vi "fgv_NtripClient_config.vi"(7 "cmd":T2, 11 "config val":T1={"Current NtripClient Account"={"id"="seoul", "pwd"="seoul", "ref pt"="YONS-RTCM32-M5", "address"="gnss.eseoul.go.kr", "port "=2101}, "Mount points"=0, "Ref r size"=1.0, "TMarr limit"=200, "Sel NMEA type"=enum."$GPGGA", "Local Time offset"=9, "Write delay ms"=900, "GNSS Serial delay"=20, "Extra Serial delay"=20, "Ntrip accounts"=[], "Send Serial config"={"NMEA out port"="COM10", "baud rate"=115200}} {"Ref r size" format="%.2f"; "Mount points" items=["SONP-RTCM32", "GANS-RTCM32", "GUMC-RTCM32", "DBON-RTCM32", "YONS-RTCM23", "SONP-RTCM23", "GUMC-RTCM23", "GANS-RTCM31", "YONS-CMRx", "SONP-RTCM31", "GUMC-RTCM31", "GANS-RTCM23", "DBON-RTCM23", "DBON-RTCM31", "YONS-RTCM31", "YONS-RTCM32-M5", "VRS-RTCM32-M5", "VRS-RTCM31", "VRS-CMRx", "VRS-CMRplus"]}) -> (3 "config val out":T1={"Current NtripClient Account"={"id"="seoul", "pwd"="seoul", "ref pt"="YONS-RTCM32-M5", "address"="gnss.eseoul.go.kr", "port "=2101}, "Mount points"=0, "Ref r size"=1.0, "TMarr limit"=200, "Sel NMEA type"=enum."$GPGGA", "Local Time offset"=9, "Write delay ms"=900, "GNSS Serial delay"=20, "Extra Serial delay"=20, "Ntrip accounts"=[], "Send Serial config"={"NMEA out port"="COM10", "baud rate"=115200}} {"Ref r size" format="%.2f"; "Mount points" items=["SONP-RTCM32", "GANS-RTCM32", "GUMC-RTCM32", "DBON-RTCM32", "YONS-RTCM23", "SONP-RTCM23", "GUMC-RTCM23", "GANS-RTCM31", "YONS-CMRx", "SONP-RTCM31", "GUMC-RTCM31", "GANS-RTCM23", "DBON-RTCM23", "DBON-RTCM31", "YONS-RTCM31", "YONS-RTCM32-M5", "VRS-RTCM32-M5", "VRS-RTCM31", "VRS-CMRx", "VRS-CMRplus"]})   [LabVIEW 2019]
uses:
  Ctrl/cmd_common.ctl
  Ctrl/GNSS-Ntrip config.ctl
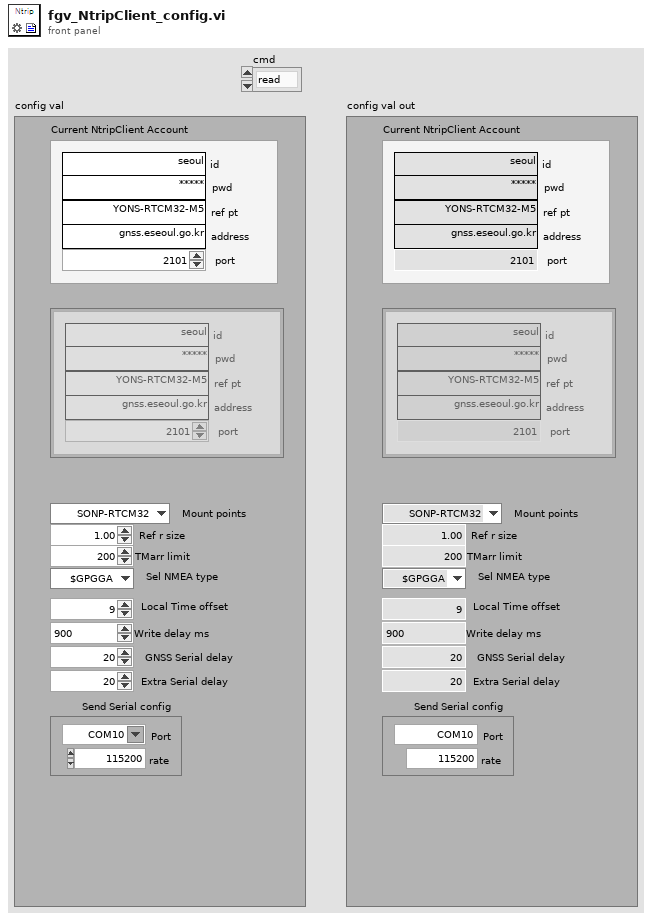
[diagram p1: front panel]
types:
  T1 = typedef "GNSS-Ntrip config.ctl" = cluster{"Current NtripClient Account":cluster{"id":string, "pwd":string, "ref pt":string, "address":string, "port ":u16}, "Mount points":u16, "Ref r size":dbl, "TMarr limit":i32, "Sel NMEA type":enum16{"$GPGSV", "$GLGSV", "$GPGGA", "$GAGSV", "$GBGSV", "$GNGLL", "$GNGGA", "$GNGSA", "$GNRMC", "$GNVTG"}, "Local Time offset":u32, "Write delay ms":u32, "GNSS Serial delay":u32, "Extra Serial delay":u32, "Ntrip accounts":cluster{"id":string, "pwd":string, "ref pt":string, "address":string, "port ":u16}[], "Send Serial config":cluster{"NMEA out port":refnum<visa-resource-name>, "baud rate":u32}}
  T2 = typedef "cmd_common.ctl" = enum16{"read", "write"}
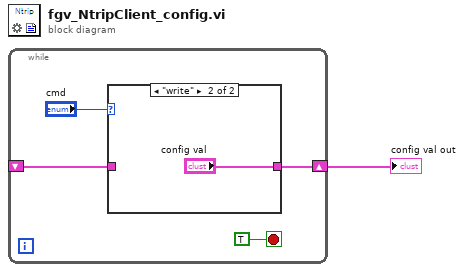
[diagram p0: block diagram]
diagram:
  n1 = while {
    shift-right: [w3] -> w1
    shift-left: _ -> [w2]
    stop <- TRUE stop-if-true
    n2 = case shown="\"write\"" "cmd" {
      tunnel: [w6 "config val"] -> w3
      tunnel: w2 -> [w6 _]
      frame "read", Default {
      }
      frame "write" {
      }
    }
  }
  "config val out" <- w1
